vi "Get_Time.vi"(1 "Index":i32, 2 "Input Sequence":cluster{string, string[], dbl[], dbl}[](array[cluster])) -> (0 "Time (s)":dbl)   [LabVIEW 2011]
doc: "This VI returns the time value associated with the event given by the \"Index\" in relation to the \"Input Sequence\"."
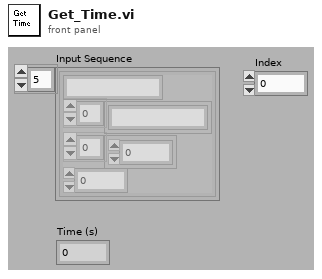
[diagram p1: front panel]
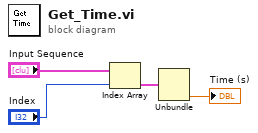
[diagram p0: block diagram]
diagram:
  n1 = Index Array(array="Input Sequence", index="Index") -> (element=w2:cluster{string, string[], dbl[], dbl})
  n2 = Unbundle(w2) -> (→"Time (s)":dbl)  [unwired: 3 out]
